vi "wait for calibration.vi"() -> ()   [LabVIEW 2012]
doc: "SciScan 1.2 160622"
uses:
  GFG/GFGfpRefGet.vi
  GFG/GFG library.lvlib
panel:
  out "String 3":string
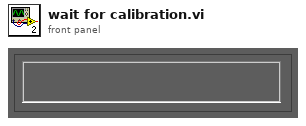
[diagram p1: front panel]
types:
  T1 = cluster{"WaveformChartRef":refnum<vi>, "DigitalRef":refnum<vi>, "ArrayRef":refnum<vi>, "TabControlRef":refnum<vi>, "EnumRef":refnum<vi>, "RingRef":refnum<vi>, "BooleanRef":refnum<vi>, "KnobRef":refnum<vi>, "SlideRef":refnum<vi>, "PathRef":refnum<vi>, "StringRef":refnum<vi>, "ComboBox":refnum<vi>, "WaveformGraphRef":refnum<vi>}
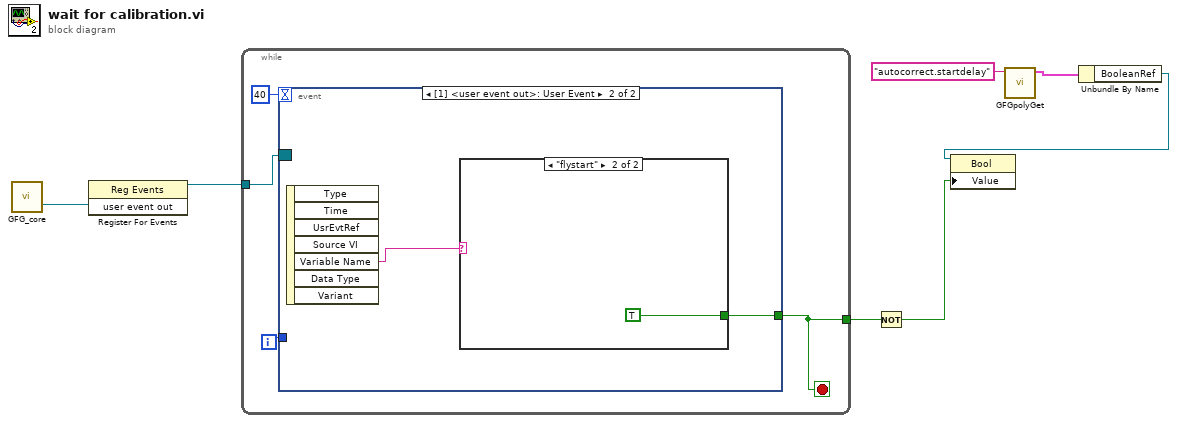
[diagram p0: block diagram]
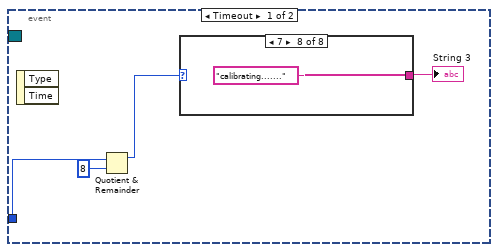
[diagram p2: hidden frame]
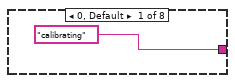
[diagram p3: hidden frame]
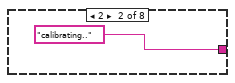
[diagram p4: hidden frame]
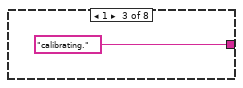
[diagram p5: hidden frame]
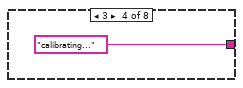
[diagram p6: hidden frame]
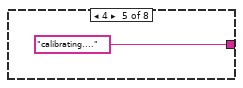
[diagram p7: hidden frame]
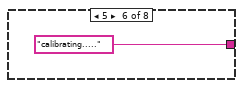
[diagram p8: hidden frame]
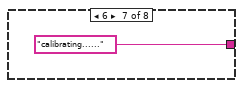
[diagram p9: hidden frame]
diagram:
  n1 = call "GFG_core.vi"() -> ("user event out"=w7:refnum<user-event>)  [unwired: 13 in, 6 out]
  n2 = register-events(w7) -> (reference out=w6:refnum<event-registration>)  [unwired: 2 in, 1 out]
  n3 = while {
    tunnel: w6 -> [w9]
    tunnel: [w8] -> w2
    i -> [w11]
    stop <- w8 stop-if-true
    n4 = event shown="[1] <user event out>: User Event" {
      selector: w9 -> [_ _]
      dyn-events: _ -> [_ _]
      timeout: 40 -> [_ _]
      tunnel: w11 -> [w14 _]
      tunnel: [_ w24] -> w8
      event Timeout {
        n5 = event-data() -> ()  [unwired: 1 in, 2 out]
        n6 = Quotient & Remainder(x=w14, y=8) -> (x-y*floor(x/y)=w12:i32)  [unwired: 1 out]
        n7 = case shown="7" w12 {
          tunnel: ["calibrating" "calibrating.." "calibrating." "calibrating..." "calibrating...." "calibrating....." "calibrating......" "calibrating......."] -> w15
          frame 0, Default {
          }
          frame 2 {
          }
          frame 1 {
          }
          frame 3 {
          }
          frame 4 {
          }
          frame 5 {
          }
          frame 6 {
          }
          frame 7 {
          }
        }
        "String 3" <- w15
      }
      event User Event {
        n8 = event-data() -> ("Variable Name"=w25:string)  [unwired: 1 in, 6 out]
        n9 = case shown="\"flystart\"" w25 {
          tunnel: [_ TRUE] -> w24
          frame "False", Default {
          }
          frame "flystart" {
          }
        }
      }
    }
  }
  n10 = Not(x=w2) -> (.not. x?=w1:bool)
  n11 = call-poly "GFGpolyGet.vi"("Variable Name in"="autocorrect.startdelay") -> ("output cluster"=w5:T1)  [unwired: 9 in, 1 out]
  n12 = Unbundle By Name(w5) -> ("BooleanRef"=w3:refnum<vi>)
  n13 = property class="Bool"(reference=w3, "Value"=w1) -> ()  [unwired: 1 in, 2 out]
